vi "Acquire Continuous Multi Echo Data.vi"(0 "VISA resource name":refnum<visa-resource-name>, 1 "Cluster Count (1)":dbl=1.0, 2 "Scan Interval (1)":dbl=1.0, 5 "Start Point (-120°)":dbl=-120.0, 7 "End Point (120°)":dbl=120.0, 9 "Number of Scans (0)":dbl, 11 "error in (no error)":errorcluster, 12 "Enable Request Message (F:Disable)":bool) -> (4 "VISA resource name out":refnum<visa-resource-name>, 6 "Magnitude Array":i32[][](array[numeric]), 8 "Direction":dbl[](array[numeric]), 10 "Scan Ended?":bool, 14 "Number of Pending Scans":i32=1, 15 "error out":errorcluster)   [LabVIEW 2014, in "Hokuyo URG Series.lvlib"]
doc: "This VI takes four parameters (start point, end point, cluster count, number of scans) and returns two arrays which describe the magnitude and angle at which the data was acquired and number of pending scans. \n\nThe reference for the angles (in the Direction array) is the center of the device which is 0° with positive angles to the left of center and negative angles to the right.\n\nThe URG-04LX can take measurements in the range of -120° to 120° and has an \"operating range\" of -135° to 135°. \n\nCluster Count refers to the number of measurements which are clustered together. \n<b>Ex:</b>If the cluster count is 3 then the smallest of three measurements is returned.\n\nScan Interval refers to the number of scans to wait (no measurement is computed) after one measurement scan is performed.\n<b>Ex:</b>the scan interval should be less than 10.\n\nNumber of Scans refers to the total number of scans for which measurement is computed.\n<b>Ex:</b>A value of 0 means unlimited scans. The number of scans should be less than 100.\n\nThe Magnitude array is associated with the Direction array. \n<b>Ex:</b> If the information for the first measurement is desired, then the 0th index of each array is accessed and returns the magnitude and direction of the first measurement.\n\nScan Ended? specifies whether the scan is over or not.\n\n\nNumber of pending scans indicates how many more scans remain to be read, not including the current message. In the very last scan response message, the number of pending scans is set to 0, and when the number of scans is unlimited, the number of pending scans in all the scan response message is also 0.\n\nIf checksums are being used and the checksum fails, the data returned in the magnitude array will default to -1."
uses:
  Hokuyo URG Series.lvlib
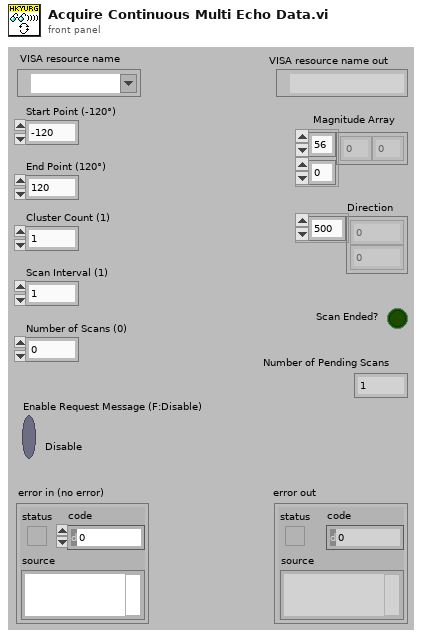
[diagram p1: front panel]
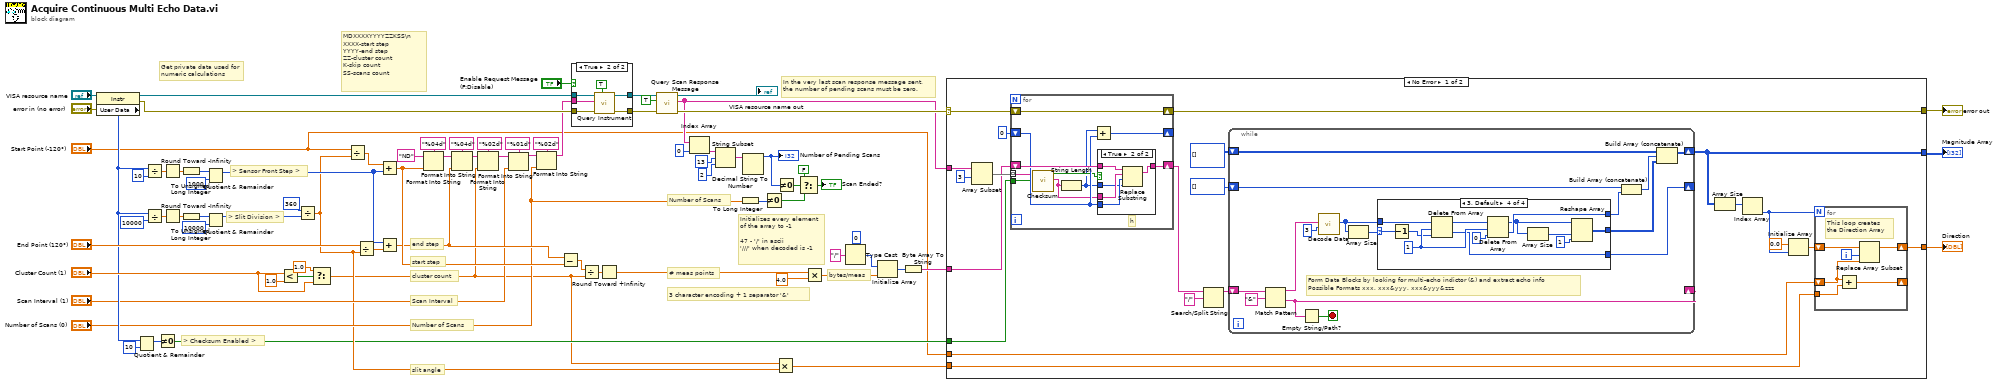
[diagram p0: block diagram]
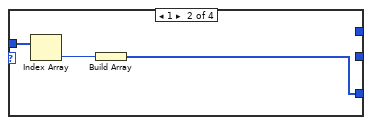
[diagram p3: hidden frame]
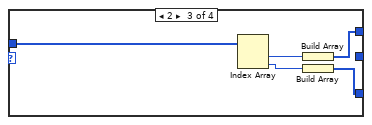
[diagram p4: hidden frame]
diagram:
  # "> Checksum Enabled >"
  # "3 character encoding + 1 separator '&'"
  # "In the very last scan response message sent,\nthe number of pending scans must be zero."
  # "Number of Scans"
  # "Number of Scans"
  # "Scan Interval"
  # "Get private data used for numeric calculations"
  # "> Slit Division >"
  # "> Sensor Front Step >"
  # "bytes/meas"
  # "# meas points"
  # "cluster count"
  # "start step"
  # "end step"
  # "slit angle"
  # "Initializes every element\nof the array to -1\n\n47 - '/' in ascii\n'///' when decoded is -1"
  # "MDXXXXYYYYZZKSS\\n\nXXXX-start step\nYYYY-end step\nZZ-cluster count\nK-skip count\nSS-scans count"
  n1 = property class="Instr"(reference="VISA resource name", error in="error in (no error)") -> (reference out=w40:refnum<visa-resource-name>, error out=w39:errorcluster, "User Data"=w42:u32)
  n2 = Quotient & Remainder(x=w42, y=u32 10) -> (x-y*floor(x/y)=w1:u32)  [unwired: 1 out]
  n3 = Divide(x=w42, y=u32 10) -> (x/y=w55:dbl)
  n4 = Divide(x=w42, y=u32 10000) -> (x/y=w49:dbl)
  n5 = Not Equal To 0?(x=w1) -> (x != 0?=w9:bool)
  n6 = Round Toward -Infinity(1:w55) -> (0:w51:dbl)
  n7 = Round Toward -Infinity(1:w49) -> (0:w48:dbl)
  n8 = To Unsigned Long Integer(number=w51) -> (unsigned 32bit integer=w54:u32)
  n9 = To Unsigned Long Integer(number=w48) -> (unsigned 32bit integer=w47:u32)
  n10 = Quotient & Remainder(x=w54, y=u32 1000) -> (x-y*floor(x/y)=w53:u32)  [unwired: 1 out]
  n11 = Quotient & Remainder(x=w47, y=u32 10000) -> (x-y*floor(x/y)=w45:u32)  [unwired: 1 out]
  n12 = Less?(x="Cluster Count (1)", y=1.0) -> (x < y?=w67:bool)
  n13 = Divide(x=u32 360 ("y"), y=w45) -> (x/y=w13:dbl)
  n14 = Select(t=1.0, s=w67, f="Cluster Count (1)") -> (s? t:f=w2:dbl)
  n15 = Divide(x="Start Point (-120°)", y=w13) -> (x/y=w64:dbl)
  n16 = Divide(x="End Point (120°)", y=w13) -> (x/y=w61:dbl)
  n17 = Add(x=w64, y=w53) -> (x+y=w63:dbl)
  n18 = Add(x=w53, y=w61) -> (x+y=w60:dbl)
  n19 = Format Into String(format string="%04d", initial string="ND", w63) -> (resulting string=w76:string)  [unwired: 1 in, 1 out]
  n20 = Format Into String(format string="%04d", initial string=w76, w60) -> (resulting string=w74:string)  [unwired: 1 in, 1 out]
  n21 = Format Into String(format string="%02d", initial string=w74, w2) -> (resulting string=w33:string)  [unwired: 1 in, 1 out]
  n22 = Format Into String(format string="%01d", initial string=w33, "Scan Interval (1)") -> (resulting string=w35:string)  [unwired: 1 in, 1 out]
  n23 = Format Into String(format string="%02d", initial string=w35, "Number of Scans (0)") -> (resulting string=w32:string)  [unwired: 1 in, 1 out]
  n24 = Subtract(x=w60, y=w63) -> (x-y=w72:dbl)
  n25 = case shown="True" "Enable Request Message (F:Disable)" {
    tunnel: w40 -> [w80 w86]
    tunnel: w39 -> [w79 w85]
    tunnel: w32 -> [_ w83]
    tunnel: [w79 w82] -> w30
    tunnel: [w80 w81] -> w29
    frame False {
    }
    frame True {
      n26 = call "Query Instrument.vi"("Error Query (Enabled)"=TRUE, "error in"=w85, "Command"=w83, "VISA Resource Name"=w86) -> ("error out"=w82:errorcluster, "VISA Resource Name Out"=w81:refnum<visa-resource-name>)  [unwired: 5 in, 1 out]
    }
  }
  n27 = Divide(x=w72, y=w2) -> (x/y=w73:dbl)
  n28 = Round Toward +Infinity(x=w73) -> (ceil(x): smallest int >= x=w70:dbl)
  n29 = call "Query Scan Response Message.vi"("error in"=w30, "Error Query (Enabled)"=TRUE, "VISA resource name"=w29) -> ("error out"=w12:errorcluster, "Response Strings"=w10:string[], "VISA resource name out"=→"VISA resource name out":refnum<visa-resource-name>)  [unwired: 6 in]
  n30 = Index Array(array=w10, index=0) -> (element=w25:string)
  n31 = String Subset(string=w25, offset (0)=13, length (rest)=2 ("length (rest)")) -> (substring=w21:string)
  n32 = To Long Integer(number="Number of Scans (0)") -> (32bit integer=w17:i32)
  n33 = Decimal String To Number(string=w21) -> (number=w15:i32)  [unwired: 2 in, 1 out]
  "Number of Pending Scans" <- w15
  n34 = Not Equal To 0?(x=w17) -> (x != 0?=w18:bool)
  n35 = Multiply(x=w2, y=w13) -> (x*y=w7:dbl)
  n36 = Not Equal To 0?(x=w15) -> (x != 0?=w20:bool)
  n37 = Select(t=FALSE, s=w20, f=w18) -> (s? t:f=→"Scan Ended?":bool)
  n38 = Multiply(x=w70, y=4.0 ("byte encoding width")) -> (x*y=w69:dbl)
  n39 = Type Cast(type=u8 0, x="/") -> (*(type *) &x=w56:u8)
  n40 = Initialize Array(w56, w69) -> (w71:u8[])
  n41 = Byte Array To String(unsigned byte array=w71) -> (string=w11:string)
  n42 = case shown="No Error" w12 {
    selector: w12 -> [w98 w165]
    tunnel: [w97 w165] -> w4
    tunnel: "Start Point (-120°)" -> [w107 _]
    tunnel: w7 -> [w106 _]
    tunnel: [w105 _] -> w6
    tunnel: w10 -> [w101 _]
    tunnel: w9 -> [w99 _]
    tunnel: w11 -> [w96 _]
    tunnel: [w90 _] -> w5
    frame No Error {
      n43 = Array Subset(array=w101, index=3 ("y")) -> (w100:string[])  [unwired: 1 in]
      n44 = for {
        shift-right: [w144] -> w97
        shift-left: w98 -> [w144]
        shift-right: [w152] -> w93
        shift-left: w96 -> [w151]
        shift-right: [w149] -> _
        shift-left: 0 -> [w150]
        tunnel: w99 -> [w147]
        tunnel: w100 -> [w143] mode=indexing
        # "h"
        n45 = call "Checksum.vi"("Checksum (Off)"=w147, "Input"=w143) -> ("Data Buffer"=w146:string, "Checksum Pass?"=w148:bool)  [unwired: 8 out]
        n46 = String Length(string=w146) -> (length=w145:i32)
        n47 = Add(x=w145, y=w150) -> (x+y=w149:i32)
        n48 = case shown="True" w148 {
          tunnel: [w153 w154] -> w152
          tunnel: w151 -> [w153 w158]
          tunnel: w146 -> [_ w157]
          tunnel: w150 -> [_ w156]
          tunnel: w145 -> [_ w155]
          frame False {
          }
          frame True {
            n49 = Replace Substring(2:w155, 3:w156, 4:w157, 5:w158) -> (1:w154:string)  [unwired: 1 out]
          }
        }
      }
      n50 = Search/Split String(string=w93, search string/char (-)="/") -> (substring before match=w91:string)  [unwired: 1 in, 2 out]
      n51 = while {
        shift-right: [w115] -> _
        shift-left: w91 -> [w122]
        shift-right: [w117] -> _
        shift-left: i32[] [] -> [w119]
        shift-right: [w116] -> w90
        shift-left: i32[][] [] -> [w112]
        stop <- w114 stop-if-true
        # "Form Data Blocks by looking for multi-echo indictor (&) and extract echo info \nPossible Formats xxx, xxx&yyy, xxx&yyy&zzz"
        n52 = Match Pattern(string=w122, regular expression="&") -> (before substring=w121:string, after substring=w115:string)  [unwired: 1 in, 2 out]
        n53 = Empty String/Path?(string/path=w115) -> (empty?=w114:bool)
        n54 = call "Decode Data.vi"("n character encoding"=u32 3, "Input Buffer"=w121) -> ("Decoded Measurements"=w120:i32[])  [unwired: 3 in, 6 out]
        n55 = Array Size(array=w120) -> (size(s)=w109:i32)
        n56 = case shown="3, Default" w109 {
          selector: w109 -> [_ _ _ w142]
          tunnel: w120 -> [_ w125 w130 w136]
          tunnel: [_ _ w128 w140] -> w118
          tunnel: [_ w123 w126 w137] -> w117
          tunnel: [_ _ _ w133] -> w110
          frame 0 {
          }
          frame 1 {
            n57 = Index Array(array=w125) -> (element=w124:i32)  [unwired: 1 in]
            n58 = Build Array(w124) -> (w123:i32[])
          }
          frame 2 {
            n59 = Index Array(array=w130) -> (element #1=w129:i32, element #2=w127:i32)  [unwired: 2 in]
            n60 = Build Array(w129) -> (w128:i32[])
            n61 = Build Array(w127) -> (w126:i32[])
          }
          frame 3, Default {
            w139 = 1 ("length")
            n62 = Decrement(x=w142) -> (x-1=w138:i32)
            n63 = Delete From Array(array=w136, length=w139, index=w138) -> (deleted portion=w137:i32[], array with subset deleted=w135:i32[])
            n64 = Delete From Array(array=w135, length=w139, index=0) -> (deleted portion=w140:i32[], array with subset deleted=w134:i32[])
            n65 = Array Size(array=w134) -> (size(s)=w132:i32)
            n66 = Reshape Array(w134, w132, 1 ("dimension size")) -> (w133:i32[][])
          }
        }
        n67 = Build Array (concatenate)(w119, w118) -> (w111:i32[])
        n68 = Build Array (concatenate)(w112, w111, w110) -> (w116:i32[][])
      }
      n69 = Array Size(array=w90) -> (size(s)=w95:i32[])
      n70 = Index Array(array=w95) -> (element=w88:i32)  [unwired: 1 in]
      n71 = Initialize Array(0.0 ("element"), w88) -> (w103:dbl[])
      n72 = for {
        N: w88 -> [_]
        shift-right: [w163] -> _
        shift-left: w107 -> [w160]
        tunnel: w106 -> [w164]
        shift-right: [w161] -> w105
        shift-left: w103 -> [w162]
        i -> [w159]
        # "This loop creates \nthe Direction Array"
        n73 = Add(x=w160, y=w164) -> (x+y=w163:dbl)
        n74 = Replace Array Subset(array=w162, new element=w160, index=w159) -> (w161:dbl[])
      }
    }
    frame Error {
    }
  }
  "error out" <- w4
  "Magnitude Array" <- w5
  "Direction" <- w6
